vi "Write U8 Array.vi"(6 "FIFO Timestamps":T1, 7 "Channel Array in":refnum<class "CIFChannels.lvclass">[](array[class]), 8 "error in (no error)":errorcluster, 9 "Data in":u8[](array[numeric]), 10 "Channel Index":i32) -> (0 "error out":errorcluster, 1 "timed out?":bool, 5 "Channel Array out":refnum<class "CIFChannels.lvclass">[](array[class]))   [LabVIEW 2021, in "CIFChannelMng.lvclass"]
uses:
  CIFChannelMng.lvclass
  <vilib>/CIF Foundation/CIF Channels Core/ChannelCommon/typedef/TimeStamps.ctl
  CIFChannelMng.lvclass/CIFChannelMng.ctl
  <vilib>/CIF Foundation/CIF Channels Core/CIFChannels/CIFChannels.lvclass
  <vilib>/CIF Foundation/CIF Channels Core/ChannelCommon/ChannelCommon.lvlib
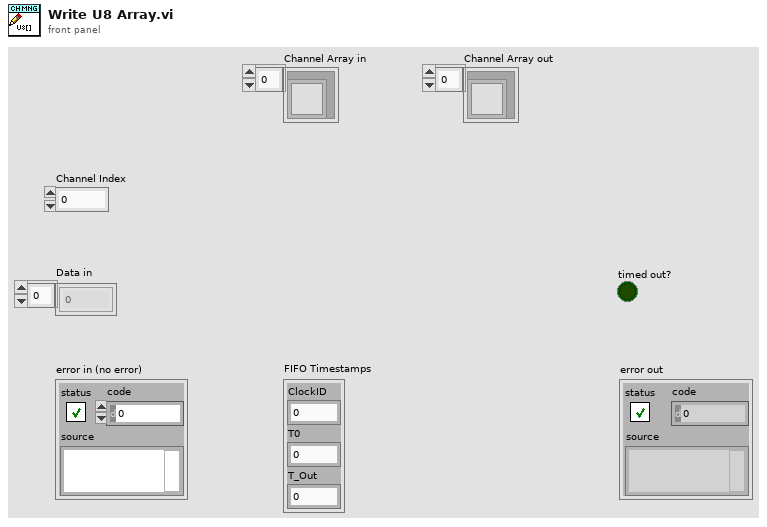
[diagram p1: front panel]
types:
  T1 = typedef "ChannelCommon.lvlib/TimeStamps.ctl" = cluster{"ClockID":u8, "T0":i64, "T_Out":i64}
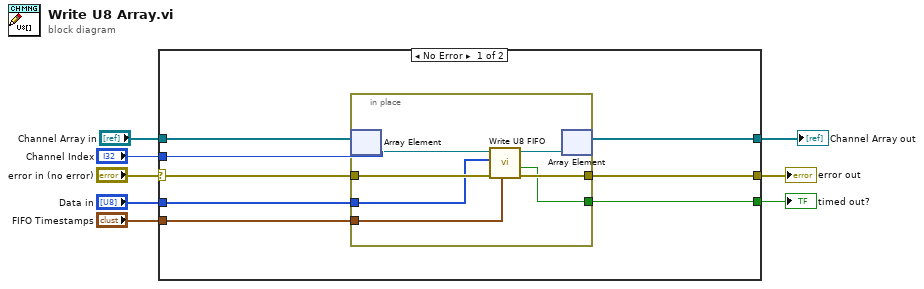
[diagram p0: block diagram]
diagram:
  n1 = case shown="No Error" "error in (no error)" {
    selector: "error in (no error)" -> [w16 w25]
    tunnel: [w15 w25] -> w7
    tunnel: [w9 w24] -> w1
    tunnel: "Channel Array in" -> [w10 w24]
    tunnel: [w14 _] -> w6
    tunnel: "Channel Index" -> [w13 _]
    tunnel: "Data in" -> [w12 _]
    tunnel: "FIFO Timestamps" -> [w11 _]
    frame No Error {
      n2 = in-place {
        in-place-border: w16 -> [w21]
        in-place-border: [w20] -> w15
        in-place-border: [w19] -> w14
        in-place-border: w12 -> [w18]
        in-place-border: w11 -> [w17]
        n3 = in-place-array #1(w10, w13) -> (w23:refnum<class "CIFChannels.lvclass">)
        n4 = call-dynamic "Write U8 FIFO.vi"("FIFO Timestamps"=w17, "error in (no error)"=w21, "Data in"=w18, "CIFChannels in"=w23) -> ("error out"=w20:errorcluster, "timed out?"=w19:bool, "CIFChannels out"=w22:refnum<class "CIFChannels.lvclass">)  [unwired: 4 in, 1 out]
        n5 = in-place-array #1(w22) -> (w9:refnum<class "CIFChannels.lvclass">[])  [unwired: 1 out]
      }
    }
    frame Error {
    }
  }
  "error out" <- w7
  "timed out?" <- w6
  "Channel Array out" <- w1
